vi "check_conn.vi"(4 "error in (no error)":errorcluster) -> (0 "error out":errorcluster, 2 "modem used":bool)   [LabVIEW 2010]
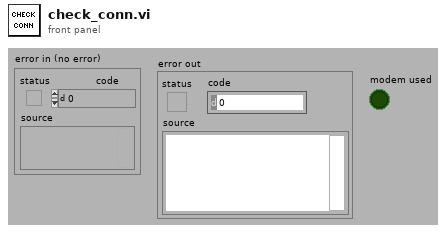
[diagram p1: front panel]
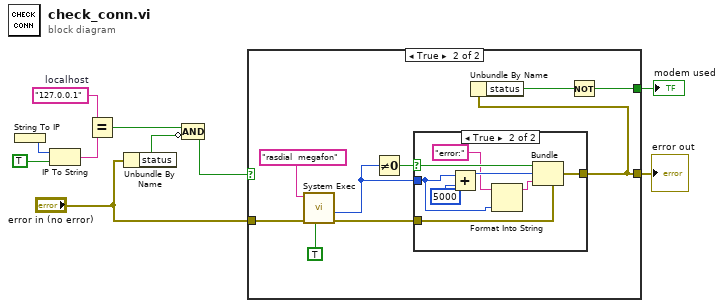
[diagram p0: block diagram]
diagram:
  w3 = "127.0.0.1"  # localhost
  n1 = String To IP() -> (0:w5:u32)  [unwired: 1 in]
  n2 = IP To String(1:TRUE ("dot notation? (F)"), 2:w5) -> (0:w2:string)
  n3 = Equal?(x=w3, y=w2) -> (x = y?=w1:bool)
  n4 = Unbundle By Name("error in (no error)") -> ("status"=w8:bool)
  n5 = Compound Arithmetic op=AND(w1, invert w8) -> (w7:bool)
  n6 = case shown="True" w7 {
    selector: w7 -> [w11 _]
    tunnel: [w12 w16] -> w10
    tunnel: "error in (no error)" -> [w12 w13]
    tunnel: [w11 w14] -> w6
    frame False {
    }
    frame True {
      n7 = call <vilib>:"System Exec.vi"("run minimized? (F)"=TRUE, "error in (no error)"=w13, "command line"="rasdial  megafon") -> ("error out"=w17:errorcluster, "return code"=w18:i32)  [unwired: 5 in, 2 out]
      n8 = Not Equal To 0?(x=w18) -> (x != 0?=w19:bool)
      n9 = case shown="True" w19 {
        selector: w19 -> [_ w30]
        tunnel: w18 -> [_ w25]
        tunnel: [w22 w27] -> w16
        tunnel: w17 -> [w22 w26]
        frame False {
        }
        frame True {
          n10 = Add(x=w25, y=5000) -> (x+y=w29:i32)
          n11 = Format Into String(initial string="error:" ("command line"), w25) -> (resulting string=w24:string)  [unwired: 2 in, 1 out]
          n12 = Bundle(cluster=w26, "status"=w30, "code"=w29, "source"=w24) -> (w27:errorcluster)
        }
      }
      n13 = Unbundle By Name(w16) -> ("status"=w15:bool)
      n14 = Not(x=w15) -> (.not. x?=w14:bool)
    }
  }
  "error out" <- w10
  "modem used" <- w6
